vi "Property - Read Config Variant.vi"(4 "error in (no error)":errorcluster, 6 "Container State":T2, 7 "Display State In":T1={"Header"="", "Label[]"=[], "DisableButtonsLUT"=variant(string[] []), "Menu Config"=variant}) -> (0 "error out":errorcluster, 2 "Value":variant, 3 "Display State Out":T1={"Header"="", "Label[]"=[], "DisableButtonsLUT"=variant(string[] []), "Menu Config"=variant})   [LabVIEW 2019, in "Menu Button.xctl"]
doc: "JSMA Module Template - Top Level UI 0.2.0.4\nRob Humfeld - Jet Engineering\nCopyright (c) 2019, Jet Engineering"
uses:
  Menu Button.xctl
  <vilib>/_xctls/Container State.ctl
  State 1.ctl
  <vilib>/_xctls/XControlSupport.lvlib
panel:
  # "Replace the Value Indicator below with an Indicator of desired type.\nDo not remove this Indicator or the others from the connector pane. \nDo not change the connector pane pattern.\nThe Value Indicator should always be the second terminal from top on the output side in the connector pane."
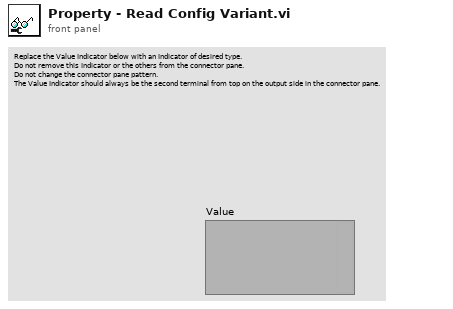
[diagram p1: front panel]
types:
  T1 = typedef "Menu Button.xctl/State 1.ctl" = cluster{"Header":string, "Label[]":string[], "DisableButtonsLUT":variant, "Menu Config":variant}
  T2 = typedef "XControlSupport.lvlib/Container State.ctl" = cluster{"Indicator?":bool, "Run Mode?":bool, " Refnum":refnum<vi>}
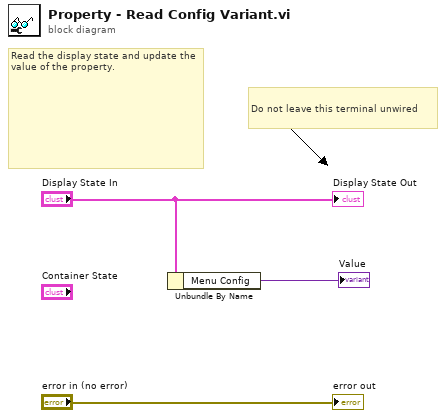
[diagram p0: block diagram]
diagram:
  # "Do not leave this terminal unwired"
  # "Read the display state and update the value of the property."
  n1 = Unbundle By Name("Display State In") -> ("Menu Config"=→"Value":variant)
  "error out" <- "error in (no error)"
  "Display State Out" <- "Display State In"
